vi "test Source Separated.vi"(8 "error in (no error)":errorcluster, 11 "TestCase in":refnum<class "Routing and Faulting Unit Tests.lvclass">) -> (0 "error out":errorcluster, 3 "TestCase out":refnum<class "Routing and Faulting Unit Tests.lvclass">)   [LabVIEW 2017, in "Routing and Faulting Unit Tests.lvclass"]
uses:
  Routing and Faulting Unit Tests.lvclass
  C:/Program Files (x86)/National Instruments/LabVIEW 2017/vi.lib/addons/_JKI Toolkits/VI Tester/TestCase.llb/TestCase.lvclass
  <vilib>/addons/_JKI Toolkits/VI Tester/TestCase.llb/TestCase.lvclass
  niveristand-custom-device-testing-tools/VeriStandTestUtilities/VeriStandTestUtilities.lvlib
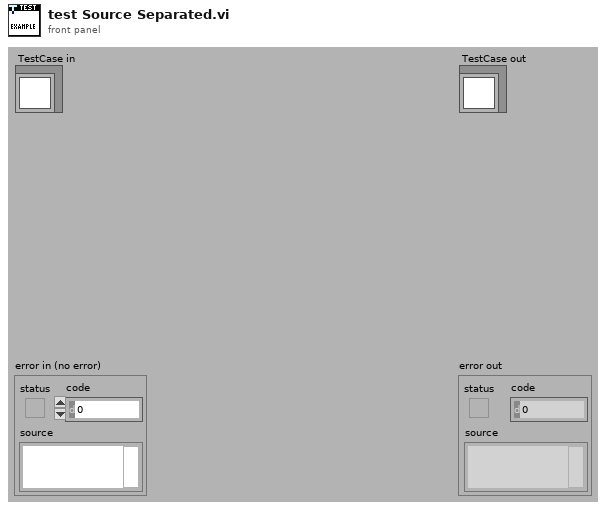
[diagram p1: front panel]
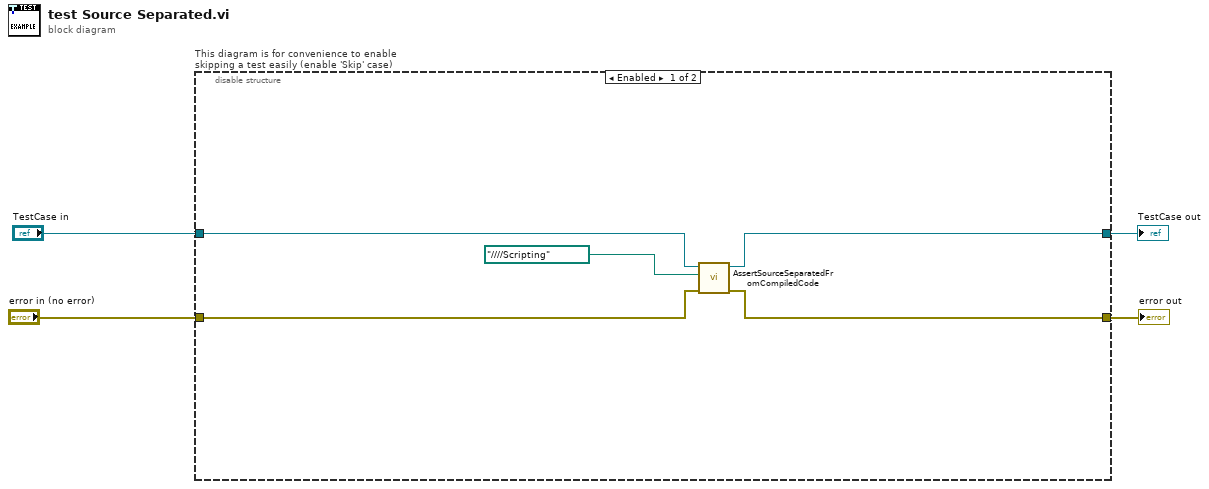
[diagram p0: block diagram]
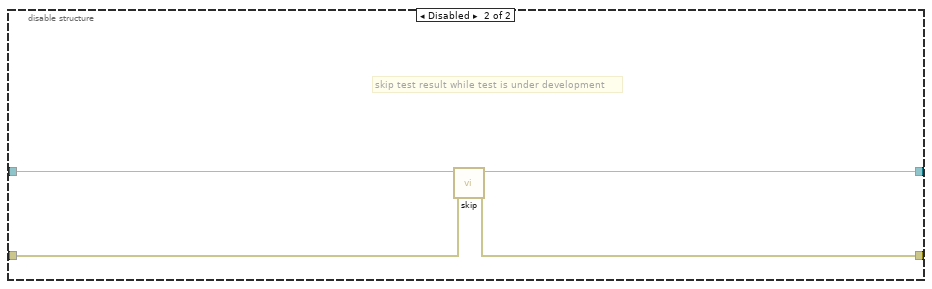
[diagram p2: hidden frame]
diagram:
  n1 = disable-structure "This diagram is for convenience to enable skipping a test easily (enable 'Skip' case)" shown="Enabled" {
    disable-tunnel: "TestCase in" -> [w9 w13]
    disable-tunnel: [w7 w11] -> w1
    disable-tunnel: [w5 w12] -> w3
    disable-tunnel: "error in (no error)" -> [w6 w10]
    frame Enabled {
      n2 = call "AssertSourceSeparatedFromCompiledCode.vi"("error in (no error)"=w6, "search path"=path "../../../../Scripting", "TestCase in"=w9) -> ("error out"=w5:errorcluster, "TestCase out"=w7:refnum<class "Routing and Faulting Unit Tests.lvclass">)  [unwired: 7 in]
    }
    frame Disabled {
      # "skip test result while test is under development"
      n3 = call <vilib>:"skip.vi"("error in (no error)"=w10, "TestCase in"=w13) -> ("error out"=w12:errorcluster, "TestCase out"=w11:refnum<class "Routing and Faulting Unit Tests.lvclass">)  [unwired: 8 in]
    }
  }
  "error out" <- w3
  "TestCase out" <- w1
